vi "DataToRead.vi"(8 "error in (no error)":errorcluster, 11 "StringReader in":refnum<class "StringReader.lvclass">) -> (0 "error out":errorcluster, 2 "Data available?":bool, 3 "StringReader out":refnum<class "StringReader.lvclass">)   [LabVIEW 2013, in "StringReader.lvclass"]
doc: "Returns TRUE if there is any data to read from the remote host"
uses:
  StringReader.lvclass
  BaseReader/BaseReader.lvclass
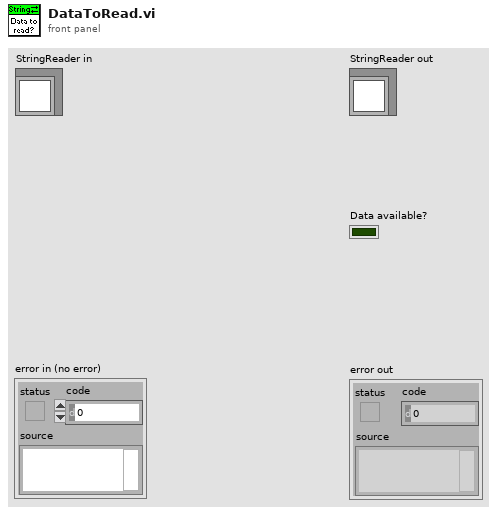
[diagram p1: front panel]
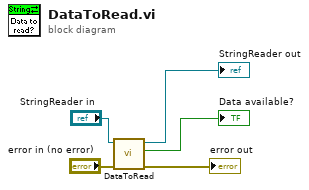
[diagram p0: block diagram]
diagram:
  n1 = call-parent "DataToRead.vi"("error in (no error)"="error in (no error)", "BaseReader in"="StringReader in") -> ("error out"=→"error out":errorcluster, "Data available?"=→"Data available?":bool, "BaseReader out"=→"StringReader out":refnum<class "StringReader.lvclass">)  [unwired: 7 in]
